vi "Controller.vi"() -> ()   [LabVIEW 2014]
uses:
  SetUp VIs/SetUp VIs.lvlib
  <vilib>/ActorFramework/Message Enqueuer/Message Enqueuer.lvclass
  Display Panel/Display Panel V3/Display Panel V3.lvclass
  Display Panel/Display Panel V3 Messages/Write String from Control Msg/Write String from Control Msg.lvclass
  Generic Instrument Messages/Send Stop Event Msg/Send Stop Event Msg.lvclass
  <vilib>/ActorFramework/Message Enqueuer/Message Priority.ctl
  <vilib>/ActorFramework/Actor/Actor.lvclass
  Subpanel Inserter Messages/Insert Into Subpanel Msg/Insert Into Subpanel Msg.lvclass
  Generic Instrument/Generic Instrument.lvclass
  Subpanel Inserter Messages/Send Stop Event Msg/Send Stop Event Msg.lvclass
panel:
  out "Output String":string
  out "Address":string
  out "Array":string[](array[string])
  out "secondary loop i":i32
  out "Display Addresses":refnum<class "Message Enqueuer.lvclass">[](array[class])
  out "error out":errorcluster
  in  "Stop Button":bool
  out "Actor Addresses":refnum<class "Message Enqueuer.lvclass">[](array[class])
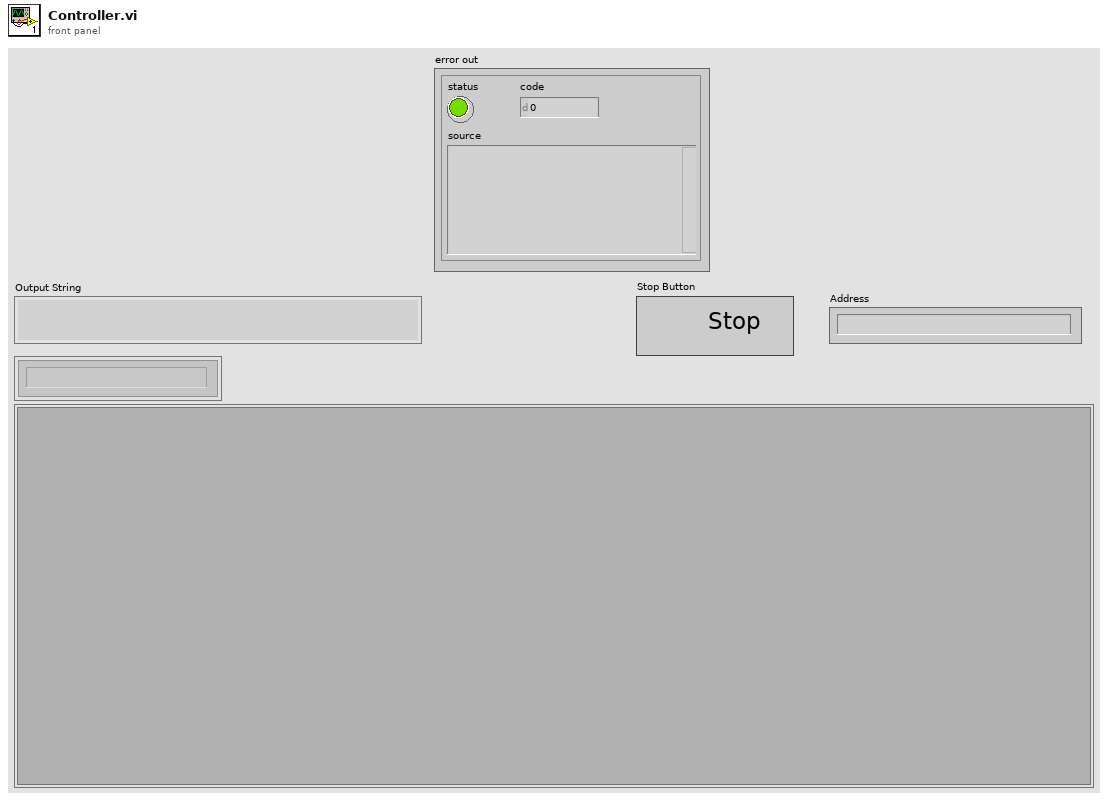
[diagram p1: front panel]
types:
  T1 = typedef "Instrument ID Object.ctl" = cluster{"Manufacturer":string, "Model":string, "Serial":string, "Address":string, "Select?":bool}
  T2 = typedef "Actor Framework.lvlib/Message Enqueuer.lvclass/Message Priority.ctl" = enum16{"Low", "Normal", "High"}
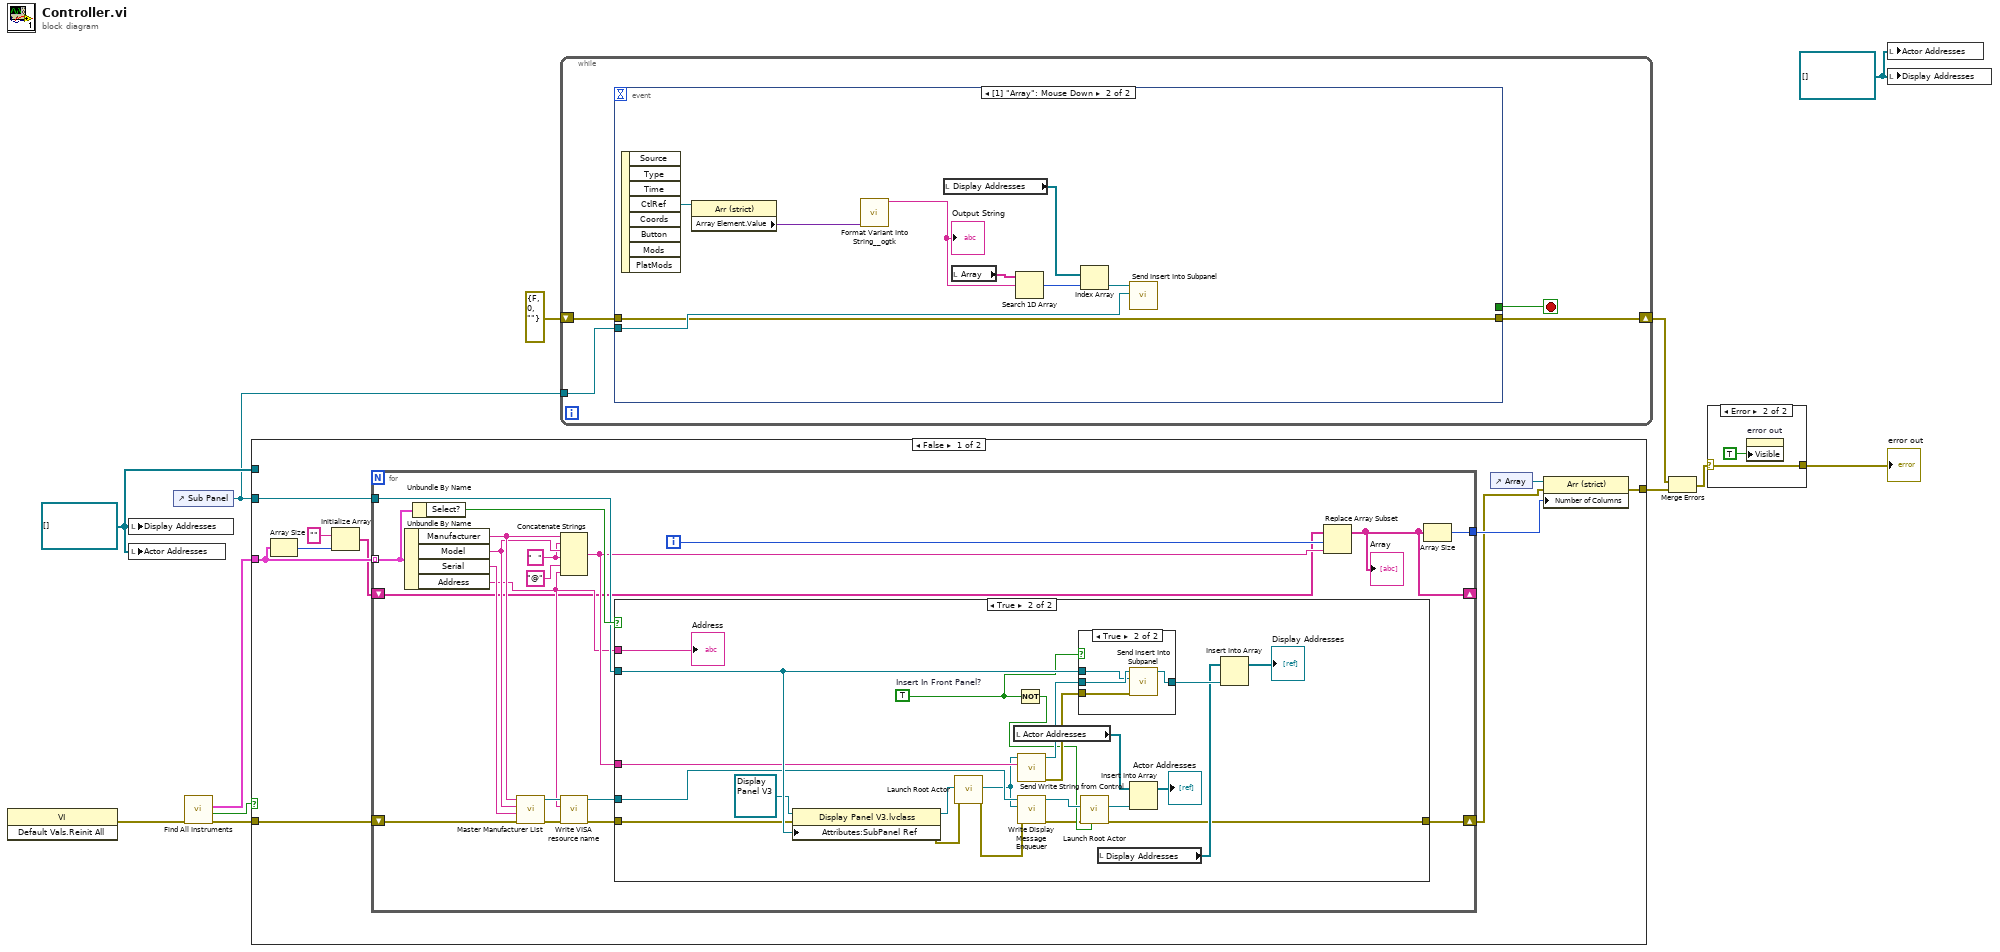
[diagram p0: block diagram]
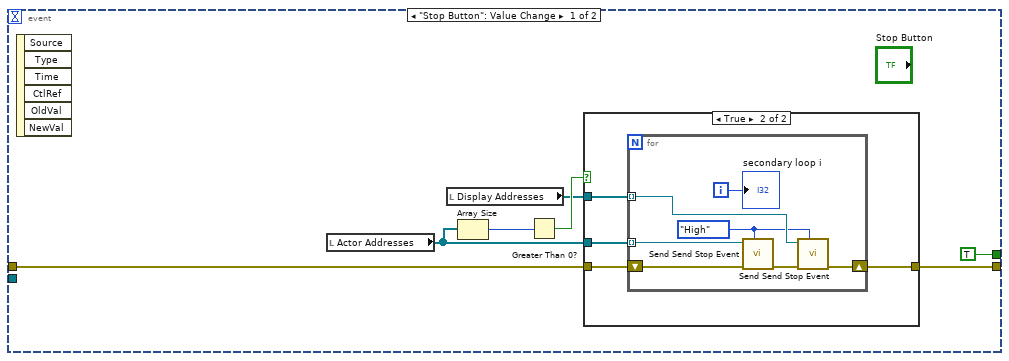
[diagram p3: hidden frame]
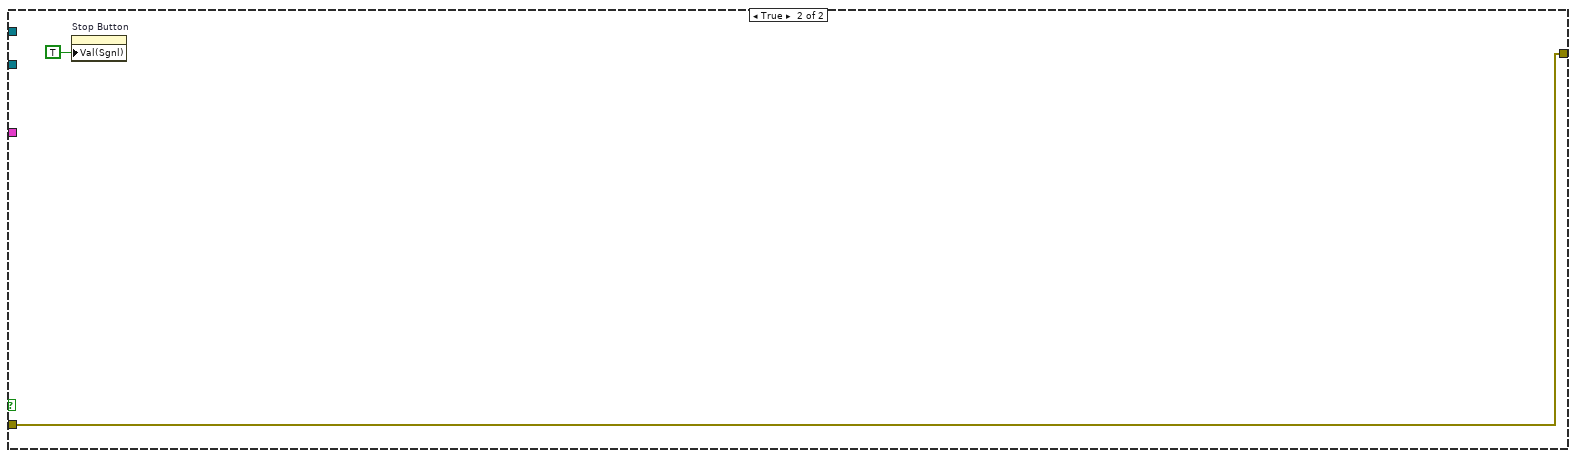
[diagram p7: hidden frame]
diagram:
  w8 = refnum<class "Message Enqueuer.lvclass">[] [] ("array")
  w10 = refnum<class "Message Enqueuer.lvclass">[] [] ("array")
  n1 = invoke class="VI" method="Default Vals.Reinit All"() -> (error out=w1:errorcluster)  [unwired: 3 in, 2 out]
  n2 = local write "Display Addresses"(w10) -> ()
  n3 = local write "Actor Addresses"(w10) -> ()
  n4 = control-ref of="Sub Panel"() -> (w7:refnum<vi>)
  n5 = call "Find All Instruments.vi"("error in (no error)"=w1) -> ("error IO"=w11:errorcluster, "Cancel Out"=w12:bool, "List of Instruments Out"=w9:T1[])  [unwired: 8 in]
  n6 = case shown="False" w12 {
    tunnel: w9 -> [w16 _]
    tunnel: w11 -> [w22 w73]
    tunnel: [w20 w73] -> w6
    tunnel: w10 -> [_ _]
    tunnel: w7 -> [w21 _]
    frame False {
      n7 = Array Size(array=w16) -> (size(s)=w18:i32)
      n8 = Initialize Array("", w18) -> (w15:string[])
      n9 = for {
        tunnel: w16 -> [w42] mode=indexing
        shift-right: [w40] -> w13
        shift-left: w22 -> [w29]
        tunnel: w21 -> [w39]
        tunnel: [w26] -> w19
        shift-right: [w23] -> _
        shift-left: w15 -> [w24]
        i -> [w27]
        w35 = "  " ("string")
        n10 = Unbundle By Name(w42) -> ("Manufacturer"=w38:string, "Model"=w36:string, "Serial"=w37:string, "Address"=w25:string)
        n11 = Unbundle By Name(w42) -> ("Select?"=w41:bool)
        n12 = call "Master Manufacturer List.vi"("error in"=w29, "Serial"=w37, "Model"=w36, "Manufacturer"=w38) -> ("error out"=w31:errorcluster, "Generic Instrument out"=w33:refnum<class "Generic Instrument.lvclass">)  [unwired: 6 in]
        n13 = Concatenate Strings(w38, w35, w36, w35, "@" ("string"), w25) -> (w28:string)
        n14 = call-dynamic "Write VISA resource name.vi"("error in (no error)"=w31, "VISA resource name"=w25, "Generic Instrument in"=w33) -> ("error out"=w30:errorcluster, "Generic Instrument out"=w32:refnum<class "Generic Instrument.lvclass">)  [unwired: 7 in]
        n15 = case shown="True" w41 {
          tunnel: w32 -> [_ w51]
          tunnel: w30 -> [w43 w50]
          tunnel: [w43 w53] -> w40
          tunnel: w39 -> [_ w62]
          tunnel: w28 -> [_ w61]
          tunnel: w25 -> [_ w59]
          frame False {
          }
          frame True {
            w56 = TRUE  # Insert In Front Panel?
            n16 = property class="Display Panel V3.lvclass"(reference=refnum<class "Display Panel V3.lvclass"> refnum ("Display Panel.lvlib:Display Panel V3.lvclass"), error in=w50, "Attributes:SubPanel Ref"=w62) -> (reference out=w44:refnum<class "Display Panel V3.lvclass">, error out=w49:errorcluster)
            n17 = call <vilib>:"Launch Root Actor.vi"("error in (no error)"=w49, "Actor"=w44) -> ("error out"=w48:errorcluster, "Actor's Enqueuer"=w46:refnum<class "Message Enqueuer.lvclass">)  [unwired: 8 in]
            n18 = local read "Actor Addresses"() -> (w58:refnum<class "Message Enqueuer.lvclass">[])
            n19 = Not(x=w56) -> (.not. x?=w52:bool)
            n20 = call "Send Write String from Control.vi"("String"=w61, "Message Enqueuer"=w46) -> ("error out"=w60:errorcluster, "Message Enqueuer out"=w64:refnum<class "Message Enqueuer.lvclass">)  [unwired: 8 in]
            n21 = call-dynamic "Write Display Message Enqueuer.vi"("error in (no error)"=w48, "Actor Framework.lvlib:Message Enqueuer"=w46, "Generic Instrument in"=w51) -> ("error out"=w47:errorcluster, "Generic Instrument out"=w55:refnum<class "Generic Instrument.lvclass">)  [unwired: 7 in]
            n22 = case shown="True" w56 {
              tunnel: w64 -> [w67 w69]
              tunnel: [w67 w71] -> w63
              tunnel: w62 -> [_ w68]
              tunnel: w60 -> [_ w70]
              frame False {
              }
              frame True {
                n23 = call "Send Insert Into Subpanel.vi"("error in (no error)"=w70, "SubPanel Ref"=w68, "Message Enqueuer"=w69) -> ("Message Enqueuer out"=w71:refnum<class "Message Enqueuer.lvclass">)  [unwired: 7 in, 1 out]
              }
            }
            n24 = call <vilib>:"Launch Root Actor.vi"("Open Actor Core front panel? (F)"=w52, "error in (no error)"=w47, "Actor"=w55) -> ("error out"=w53:errorcluster, "Actor's Enqueuer"=w54:refnum<class "Message Enqueuer.lvclass">)  [unwired: 7 in]
            n25 = local read "Display Addresses"() -> (w57:refnum<class "Message Enqueuer.lvclass">[])
            n26 = Insert Into Array(array=w58, new element=w54) -> (→"Actor Addresses":refnum<class "Message Enqueuer.lvclass">[])  [unwired: 1 in]
            n27 = Insert Into Array(array=w57, new element=w63) -> (→"Display Addresses":refnum<class "Message Enqueuer.lvclass">[])  [unwired: 1 in]
            "Address" <- w59
          }
        }
        n28 = Replace Array Subset(array=w24, new element=w28, index=w27) -> (w23:string[])
        "Array" <- w23
        n29 = Array Size(array=w23) -> (size(s)=w26:i32)
      }
      n30 = control-ref of="Array"() -> (w14:refnum<vi>)
      n31 = property class="Arr (strict)"(reference=w14, error in=w13, "Number of Columns"=w19) -> (error out=w20:errorcluster)  [unwired: 1 out]
    }
    frame True {
      n32 = property on="Stop Button" class="Bool (strict)"("Val(Sgnl)"=TRUE ("Stop Button")) -> ()  [unwired: 2 in, 2 out]
    }
  }
  n33 = while {
    tunnel: w7 -> [w76]
    shift-right: [w75] -> w4
    shift-left: errorcluster {"status"=FALSE, "code"=0, "source"=""} ("error out") -> [w74]
    stop <- w77 stop-if-true
    n34 = event shown="[1] \"Array\": Mouse Down" {
      selector: _ -> [_ _]
      dyn-events: _ -> [_ _]
      timeout: _ -> [_ _]
      tunnel: [w84 w97] -> w75
      tunnel: [TRUE _] -> w77
      tunnel: w76 -> [_ w99]
      tunnel: w74 -> [w78 w97]
      event "Stop Button": Value Change {
        n35 = event-data() -> ()  [unwired: 1 in, 6 out]
        n36 = local read "Actor Addresses"() -> (w83:refnum<class "Message Enqueuer.lvclass">[])
        n37 = local read "Display Addresses"() -> (w80:refnum<class "Message Enqueuer.lvclass">[])
        n38 = Array Size(array=w83) -> (size(s)=w82:i32)
        n39 = Greater Than 0?(x=w82) -> (x > 0?=w81:bool)
        n40 = case shown="True" w81 {
          tunnel: [w85 w89] -> w84
          tunnel: w83 -> [_ w88]
          tunnel: w80 -> [_ w87]
          tunnel: w78 -> [w85 w86]
          frame False {
          }
          frame True {
            n41 = for {
              tunnel: w88 -> [w95] mode=indexing
              shift-right: [w92] -> w89
              shift-left: w86 -> [w94]
              tunnel: w87 -> [w91] mode=indexing
              i -> [w96]
              w90 = Message_Priority."High" ("Message Priority (Normal)")
              n42 = call "Send Send Stop Event.vi"("Message Priority (Normal)"=w90, "error in (no error)"=w94, "Message Enqueuer"=w95) -> ("error out"=w93:errorcluster)  [unwired: 7 in, 1 out]
              n43 = call "Send Send Stop Event.vi"("Message Priority (Normal)"=w90, "error in (no error)"=w93, "Message Enqueuer"=w91) -> ("error out"=w92:errorcluster)  [unwired: 7 in, 1 out]
              "secondary loop i" <- w96
            }
          }
        }
      }
      event "Array": Mouse Down {
        n44 = event-data() -> ("CtlRef"=w105:refnum<vi>)  [unwired: 1 in, 7 out]
        n45 = property class="Arr (strict)"(reference=w105) -> ("Array Element.Value"=w104:variant)  [unwired: 1 in, 2 out]
        n46 = call <userlib>:"Format Variant Into String__ogtk.vi"("Variant"=w104) -> ("Output String"=w102:string)  [unwired: 13 in, 1 out]
        "Output String" <- w102
        n47 = local read "Display Addresses"() -> (w101:refnum<class "Message Enqueuer.lvclass">[])
        n48 = local read "Array"() -> (w103:string[])
        n49 = Search 1D Array(1D array=w103, element=w102) -> (index of element=w100:i32)  [unwired: 1 in]
        n50 = Index Array(array=w101, index=w100) -> (element=w98:refnum<class "Message Enqueuer.lvclass">)
        n51 = call "Send Insert Into Subpanel.vi"("SubPanel Ref"=w99, "Message Enqueuer"=w98) -> ()  [unwired: 8 in, 2 out]
      }
    }
  }
  n52 = Merge Errors(w4, w6) -> (w3:errorcluster)
  n53 = case shown="Error" w3 {
    selector: w3 -> [w106 w108]
    tunnel: [w106 w108] -> w2
    frame No Error {
    }
    frame Error {
      n54 = property on="error out" class="Clust (strict)"("Visible"=TRUE) -> ()  [unwired: 2 in, 2 out]
    }
  }
  "error out" <- w2
  n55 = local write "Actor Addresses"(w8) -> ()
  n56 = local write "Display Addresses"(w8) -> ()
